vi "Miscellaneous_Initialization.vi"   [LabVIEW 2018]
uses:
  <vilib>/Rock Robotics/WPI/Joystick/WPI_JoystickDeviceEnum.ctl
  Subsytems/Drive/Drive_Notifier.ctl
  Subsytems/Drive/Drive_Control_Type.ctl
  Subsytems/Elevator/Elevator_Notifier.ctl
  Subsytems/Elevator/Elevator_Control_Type.ctl
  Subsytems/Elevator/Elevator_Enum_States.ctl
  Subsytems/Intake_Joint/Intake_Joint_Notifier.ctl
  Subsytems/Intake_Joint/Intake_Joint_Control_Type.ctl
  Subsytems/Intake_Joint/Intake_Joint_Enum_States.ctl
  Subsytems/Intake_Ball/Intake_Ball_Notifier.ctl
  Subsytems/Intake_Ball/Intake_Ball_Control_Type.ctl
  Subsytems/Intake_Disc/Intake_Disc_Notifier.ctl
  Subsytems/Intake_Disc/Intake_Disc_Control_Type.ctl
  <vilib>/Rock Robotics/WPI/Solenoid/WPI_SolenoidValue.ctl
  Subsytems/Climb/Climb_Notifier.ctl
  Subsytems/Climb/Climb_Control_Type.ctl
  <vilib>/Rock Robotics/SystemInterfaces/DIO/FPGA_DIOPWMChannel.ctl
  Global_Variables/Drive_Globals.vi
  Global_Variables/Refnum_Names.vi
  Global_Variables/Elevator_Globals.vi
  Global_Variables/Intake_Joint_Globals.vi
  Global_Variables/Intake_Ball_Globals.vi
  Global_Variables/Intake_Disc_Globals.vi
  Global_Variables/Climb_Globals.vi
  Global_Variables/LED_Globals.vi
types:
  T1 = typedef "FPGA_DIOPWMChannel.ctl" = enum8{"PWM 0", "PWM 1", "PWM 2", "PWM 3", "PWM 4", "PWM 5", "PWM 6", "PWM 7", "PWM 8", "PWM 9", "PWM MXP 0", "PWM MXP 1", "PWM MXP 2", "PWM MXP 3", "PWM MXP 4", "PWM MXP 5", "PWM MXP 6", "PWM MXP 7", "PWM MXP 8", "PWM MXP 9", "Invalid"}
  T2 = typedef "Climb_Notifier.ctl" = cluster{"Climb_Control_Type":T3, "Brake":bool, "Manual_Climb_Up":bool, "Manual_Drive_Forward":bool, "Manual_Drive_Backward":bool, "Manual_Climb_Down":bool, "Climb_Advance":bool, "Climb_Reverse":bool, "Parameter_One":dbl, "Parameter_Two":dbl, "Parameter_Three":dbl, "Step":i32, "Climb_Notifier":refnum<notifier>, "Climb_Distance":dbl, "Level_Two":bool, "Brake_State":bool, "Toggle_Servo":bool, "Drop_Back":bool}
  T3 = typedef "Climb_Control_Type.ctl" = enum16{"No_Op", "Brake", "Manual_Climb_Up", "Manual_Climb_Down", "Manual_Drive_Forward", "Manual_Drive_Backward", "Back_Wheels_Forward", "Lift_Retract", "Lift_Extend", "Extend_to_Second_Level", "Drop_Down", "Spin"}
  T4 = typedef "Intake_Disc_Notifier.ctl" = cluster{"Intake_Disc_Control_Type":T5, "Manual_Disc_Toggle":bool, "Disc_Toggle":bool, "Disc_Toggle_State":bool, "Manual_Press_Toggle":bool, "Disc_Press_State":bool, "Press_Toggle":bool, "Press_Pnuematic":T6, "Disc_Pnuematic":T6, "Disc_Notifier":refnum<notifier>, "Step":i32}
  T5 = typedef "Intake_Disc_Control_Type.ctl" = enum16{"No_Op", "Manual_Disc_Toggle", "Disc_Toggle", "Manual_Press_Toggle", "Press_Toggle", "Acquire_Hatch", "Retract"}
  T6 = typedef "WPI_SolenoidValue.ctl" = enum16{"Off", "On", "Forward", "Reverse"}
  T7 = typedef "Intake_Ball_Notifier.ctl" = cluster{"Intake_Ball_Control_Type":T8, "Manual_In":bool, "Manual_Out":bool, "Ball_In":bool, "Ball_Out":bool, "Parameter_One":dbl, "Parameter_Two":dbl, "Parameter_Three":dbl, "Step":i32, "Ball_Notifier":refnum<notifier>}
  T8 = typedef "Intake_Ball_Control_Type.ctl" = enum16{"No_Op", "Manual_In", "Manual_Out", "In_Sensor_Stop", "Out_Teleop", "Out", "Stall"}
  T9 = typedef "Intake_Joint_Notifier.ctl" = cluster{"Intake_Joint_Control_Type":T10, "Manual_Joint_Up":bool, "Manual_Joint_Down":bool, "Low_Rocket":bool, "Mid_Rocket":bool, "High_Rocket":bool, "Cargo_Ship":bool, "Hatch_Floor":bool, "Cargo_Floor":bool, "HP_Hatch":bool, "HP_Cargo":bool, "Depot_Cargo":bool, "Stow":bool, "Intake_Mode":bool, "Set Position":T11, "Parameter_One":dbl, "Parameter_Two":dbl, "Parameter_Three":dbl, "Step":i32, "Joint_Notifier":refnum<notifier>}
  T10 = typedef "Intake_Joint_Control_Type.ctl" = enum16{"No_Op", "Manual_Joint_Up", "Manual_Joint_Down", "Manual_Position_Control", "Position_Control", "Position"}
  T11 = typedef "Intake_Joint_Enum_States.ctl" = enum16{"Current_Position", "High_Rocket_Hatch_Panel_Floor", "High_Rocket_Hatch_Panel", "Mid_Rocket_Hatch_Panel_Floor", "Mid_Rocket_Hatch_Panel", "Low_Rocket_Hatch_Panel", "Cargo_Ship_Hatch_Panel", "Loading_Station_Hatch_Panel", "Ground_Pickup_Hatch_Panel", "High_Rocket_Cargo", "Mid_Rocket_Cargo", "Low_Rocket_Cargo", "Cargo_Ship_Cargo", "Loading_Station_Cargo", "Ground_Pickup_Cargo", "Depot_Pickup_Cargo", "Stow_Cargo", "Get_Hatch"}
  T12 = typedef "Elevator_Notifier.ctl" = cluster{"Elevator_Control_Type":T13, "Shift":bool, "Brake":bool, "Manual_Lift_Up":bool, "Manual_Lift_Down":bool, "Climb_Advance":bool, "Climb_Reverse":bool, "Low_Rocket":bool, "Mid_Rocket":bool, "High_Rocket":bool, "Cargo_Ship":bool, "Hatch_Floor":bool, "Cargo_Floor":bool, "HP_Hatch":bool, "HP_Cargo":bool, "Depot_Cargo":bool, "Stow":bool, "Set_Position":T14, "Intake_Mode":bool, "Climb_Distance":dbl, "Level_Two":bool, "Parameter_One":dbl, "Parameter_Two":dbl, "Parameter_Three":dbl, "Step":i32, "Elevator_Notifier":refnum<notifier>, "Brake_State":bool, "Shift_State":bool}
  T13 = typedef "Elevator_Control_Type.ctl" = enum16{"No_Op", "Shift", "Brake", "Manual_Elevator_Up", "Manual_Elevator_Down", "Manual_Climb_Up", "Manual_Climb_Down", "Manual_Position_Control", "Elevator_Retract", "Elevator_Extend", "Brake_In_Climb", "Position_Control", "Position", "Shift_Climb"}
  T14 = typedef "Elevator_Enum_States.ctl" = enum16{"Current_Position", "High_Rocket_Hatch_Panel_Floor", "High_Rocket_Hatch_Panel", "Mid_Rocket_Hatch_Panel_Floor", "Mid_Rocket_Hatch_Panel", "Low_Rocket_Hatch_Panel", "Cargo_Ship_Hatch_Panel", "Loading_Station_Hatch_Panel", "Ground_Pickup_Hatch_Panel", "High_Rocket_Cargo", "Mid_Rocket_Cargo", "Low_Rocket_Cargo", "Cargo_Ship_Cargo", "Loading_Station_Cargo", "Ground_Pickup_Cargo", "Depot_Pickup_Cargo", "Descend_Off_Platform", "Stow_Cargo"}
  T15 = typedef "Drive_Notifier.ctl" = cluster{"Drive Control List":T16, "Front/Back":dbl, "Left/Right":dbl, "Turn":dbl, "Test_Joy_Y":dbl, "Test_Joy_X":dbl, "Set Wheel Encoder Positions":bool, "Robotcentric":bool, "Reset Gyro":bool, "Rotate Front Right":bool, "Rotate Front Left":bool, "Rotate Back Right":bool, "Rotate Back Left":bool, "Write_Encoder_Positions":bool, "Climb_Advance":bool, "Parameter_One":dbl, "Parameter_Two":dbl, "Parameter_Three":dbl, "Parameter_Four":dbl, "Drive_Notifier":refnum<notifier>, "Step":i32, "Climb_Reverse":bool, "Auto_Target":bool}
  T16 = typedef "Drive_Control_Type.ctl" = enum16{"No_Op", "Write_FL_Position", "Write_FR_Position", "Write_BL_Position", "Write_BR_Position", "Set_Encoder_Positions", "Fieldcentric_PercentVBus", "Fieldcentric", "Robotcentric", "Reset_Gyro", "FR_Wheel", "FL_Wheel", "BR_Wheel", "BL_Wheel", "Drive_Onto_Platform", "Manual_Wheel_Control", "Distance", "Turn_To_Heading", "Turn_To_Target", "Drive_To_Target", "Zero", "Auto_Target", "Drive_Over_Platform", "Heading_Lock", "Time"}
  T17 = typedef "WPI_JoystickDeviceEnum.ctl" = enum16{"USB 0", "USB 1", "USB 2", "USB 3", "USB 4", "USB 5"}
  T18 = typedef "WPI_JoystickDevRef.ctl" = cluster{"Device":T17}
  T19 = typedef "CTRE_CANifier_DeviceRef.ctl" = cluster{"DeviceStatus":errorcluster, "Device Number":u8, "Handle":u64, "UsageFrame":u32, "Library Path":path}
  T20 = typedef "WPI_ServoDeviceRef.ctl" = cluster{"DeviceStatus":errorcluster, "PWM Channel":T1, "DeadBand":T21}
  T21 = typedef "WPI_PWMDeadband.ctl" = cluster{"Name":string, "maxPositivePwm":i32, "minPositivePwm":i32, "centerPwm":i32, "maxNegativePwm":i32, "minNegativePwm":i32, "angularRange":u16}
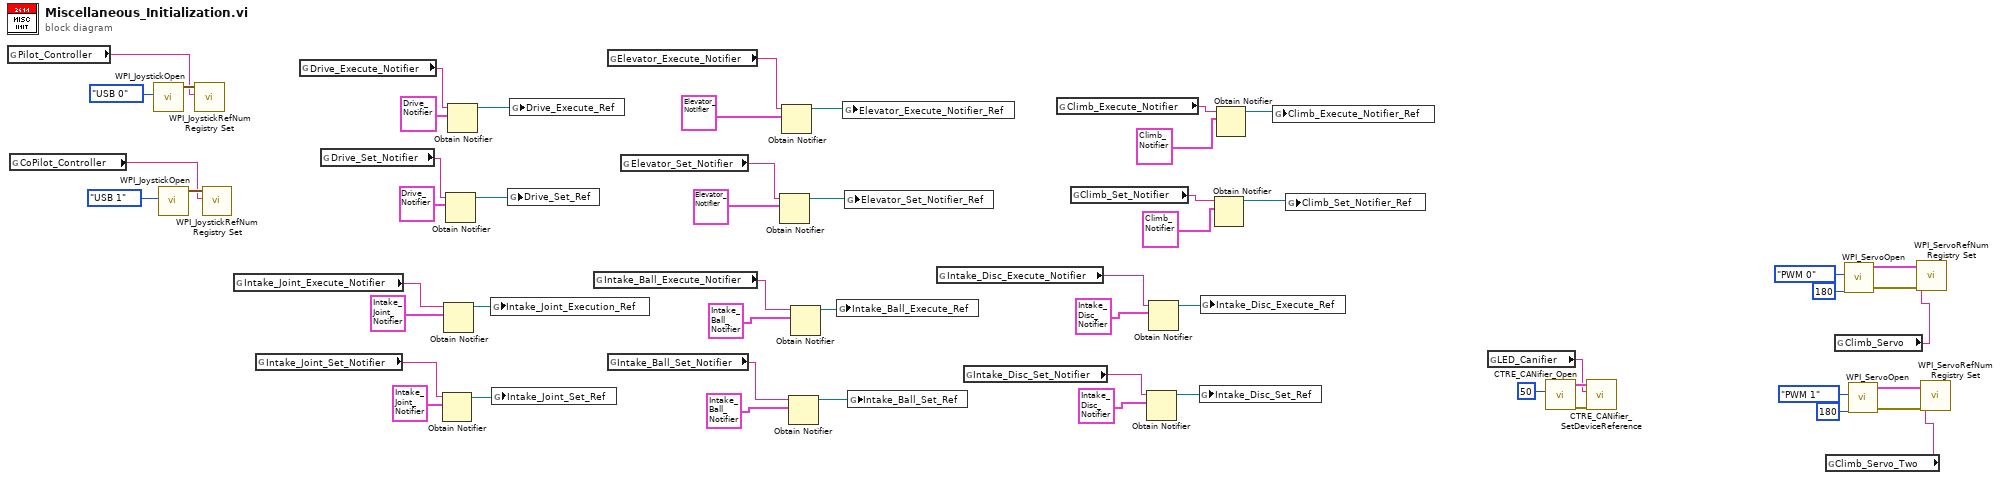
[diagram p0: block diagram]
diagram:
  n1 = global read "Refnum_Names.vi" "Pilot_Controller"() -> (w46:string)
  n2 = global read "Refnum_Names.vi" "CoPilot_Controller"() -> (w45:string)
  n3 = call <vilib>:"WPI_JoystickOpen.vi"("JoystickDevice"=WPI_JoystickDeviceEnum."USB 0") -> ("JoystickDevRef"=w56:T18)  [unwired: 10 in]
  n4 = call <vilib>:"WPI_JoystickOpen.vi"("JoystickDevice"=WPI_JoystickDeviceEnum."USB 1") -> ("JoystickDevRef"=w53:T18)  [unwired: 10 in]
  n5 = call <vilib>:"WPI_JoystickRefNum Registry Set.vi"("refnum name"=w46, "JoystickDevRef"=w56) -> ()  [unwired: 8 in, 2 out]
  n6 = call <vilib>:"WPI_JoystickRefNum Registry Set.vi"("refnum name"=w45, "JoystickDevRef"=w53) -> ()  [unwired: 8 in, 2 out]
  n7 = global read "Intake_Joint_Globals.vi" "Intake_Joint_Execute_Notifier"() -> (w36:string)
  n8 = global read "Intake_Joint_Globals.vi" "Intake_Joint_Set_Notifier"() -> (w35:string)
  n9 = global read "Drive_Globals.vi" "Drive_Execute_Notifier"() -> (w50:string)
  n10 = global read "Drive_Globals.vi" "Drive_Set_Notifier"() -> (w51:string)
  n11 = Obtain Notifier(name (unnamed)=w35, notification data type=T9 {"Intake_Joint_Control_Type"=enum."No_Op", "Manual_Joint_Up"=FALSE, "Manual_Joint_Down"=FALSE, "Low_Rocket"=FALSE, "Mid_Rocket"=FALSE, "High_Rocket"=FALSE, "Cargo_Ship"=FALSE, "Hatch_Floor"=FALSE, "Cargo_Floor"=FALSE, "HP_Hatch"=FALSE, "HP_Cargo"=FALSE, "Depot_Cargo"=FALSE, "Stow"=FALSE, "Intake_Mode"=FALSE, "Set Position"=enum."High_Rocket_Hatch_Panel", "Parameter_One"=0.0, "Parameter_Two"=0.0, "Parameter_Three"=0.0, "Step"=0, "Joint_Notifier"=refnum} ("Intake_Joint_Notifier")) -> (notifier out=w33:refnum<notifier>)  [unwired: 2 in, 2 out]
  n12 = Obtain Notifier(name (unnamed)=w36, notification data type=T9 {"Intake_Joint_Control_Type"=enum."No_Op", "Manual_Joint_Up"=FALSE, "Manual_Joint_Down"=FALSE, "Low_Rocket"=FALSE, "Mid_Rocket"=FALSE, "High_Rocket"=FALSE, "Cargo_Ship"=FALSE, "Hatch_Floor"=FALSE, "Cargo_Floor"=FALSE, "HP_Hatch"=FALSE, "HP_Cargo"=FALSE, "Depot_Cargo"=FALSE, "Stow"=FALSE, "Intake_Mode"=FALSE, "Set Position"=enum."High_Rocket_Hatch_Panel", "Parameter_One"=0.0, "Parameter_Two"=0.0, "Parameter_Three"=0.0, "Step"=0, "Joint_Notifier"=refnum} ("Intake_Joint_Notifier")) -> (notifier out=w34:refnum<notifier>)  [unwired: 2 in, 2 out]
  n13 = Obtain Notifier(name (unnamed)=w51, notification data type=T15 {"Drive Control List"=enum."No_Op", "Front/Back"=0.0, "Left/Right"=0.0, "Turn"=0.0, "Test_Joy_Y"=0.0, "Test_Joy_X"=0.0, "Set Wheel Encoder Positions"=FALSE, "Robotcentric"=FALSE, "Reset Gyro"=FALSE, "Rotate Front Right"=FALSE, "Rotate Front Left"=FALSE, "Rotate Back Right"=FALSE, "Rotate Back Left"=FALSE, "Write_Encoder_Positions"=FALSE, "Climb_Advance"=FALSE, "Parameter_One"=0.0, "Parameter_Two"=0.0, "Parameter_Three"=0.0, "Parameter_Four"=0.0, "Drive_Notifier"=refnum, "Step"=0, "Climb_Reverse"=FALSE, "Auto_Target"=FALSE} ("Drive Notifier")) -> (notifier out=w49:refnum<notifier>)  [unwired: 2 in, 2 out]
  n14 = Obtain Notifier(name (unnamed)=w50, notification data type=T15 {"Drive Control List"=enum."No_Op", "Front/Back"=0.0, "Left/Right"=0.0, "Turn"=0.0, "Test_Joy_Y"=0.0, "Test_Joy_X"=0.0, "Set Wheel Encoder Positions"=FALSE, "Robotcentric"=FALSE, "Reset Gyro"=FALSE, "Rotate Front Right"=FALSE, "Rotate Front Left"=FALSE, "Rotate Back Right"=FALSE, "Rotate Back Left"=FALSE, "Write_Encoder_Positions"=FALSE, "Climb_Advance"=FALSE, "Parameter_One"=0.0, "Parameter_Two"=0.0, "Parameter_Three"=0.0, "Parameter_Four"=0.0, "Drive_Notifier"=refnum, "Step"=0, "Climb_Reverse"=FALSE, "Auto_Target"=FALSE} ("Drive Notifier")) -> (notifier out=w52:refnum<notifier>)  [unwired: 2 in, 2 out]
  n15 = global write "Intake_Joint_Globals.vi" "Intake_Joint_Execution_Ref"(w34) -> ()
  n16 = global write "Intake_Joint_Globals.vi" "Intake_Joint_Set_Ref"(w33) -> ()
  n17 = global write "Drive_Globals.vi" "Drive_Set_Ref"(w49) -> ()
  n18 = global write "Drive_Globals.vi" "Drive_Execute_Ref"(w52) -> ()
  n19 = global read "Intake_Ball_Globals.vi" "Intake_Ball_Execute_Notifier"() -> (w32:string)
  n20 = global read "Elevator_Globals.vi" "Elevator_Execute_Notifier"() -> (w44:string)
  n21 = global read "Intake_Ball_Globals.vi" "Intake_Ball_Set_Notifier"() -> (w31:string)
  n22 = global read "Elevator_Globals.vi" "Elevator_Set_Notifier"() -> (w43:string)
  n23 = Obtain Notifier(name (unnamed)=w43, notification data type=T12 {"Elevator_Control_Type"=enum."No_Op", "Shift"=FALSE, "Brake"=FALSE, "Manual_Lift_Up"=FALSE, "Manual_Lift_Down"=FALSE, "Climb_Advance"=FALSE, "Climb_Reverse"=FALSE, "Low_Rocket"=FALSE, "Mid_Rocket"=FALSE, "High_Rocket"=FALSE, "Cargo_Ship"=FALSE, "Hatch_Floor"=FALSE, "Cargo_Floor"=FALSE, "HP_Hatch"=FALSE, "HP_Cargo"=FALSE, "Depot_Cargo"=FALSE, "Stow"=FALSE, "Set_Position"=enum."High_Rocket_Hatch_Panel", "Intake_Mode"=FALSE, "Climb_Distance"=0.0, "Level_Two"=FALSE, "Parameter_One"=0.0, "Parameter_Two"=0.0, "Parameter_Three"=0.0, "Step"=0, "Elevator_Notifier"=refnum, "Brake_State"=FALSE, "Shift_State"=FALSE} ("Elevator_Notifier")) -> (notifier out=w39:refnum<notifier>)  [unwired: 2 in, 2 out]
  n24 = Obtain Notifier(name (unnamed)=w44, notification data type=T12 {"Elevator_Control_Type"=enum."No_Op", "Shift"=FALSE, "Brake"=FALSE, "Manual_Lift_Up"=FALSE, "Manual_Lift_Down"=FALSE, "Climb_Advance"=FALSE, "Climb_Reverse"=FALSE, "Low_Rocket"=FALSE, "Mid_Rocket"=FALSE, "High_Rocket"=FALSE, "Cargo_Ship"=FALSE, "Hatch_Floor"=FALSE, "Cargo_Floor"=FALSE, "HP_Hatch"=FALSE, "HP_Cargo"=FALSE, "Depot_Cargo"=FALSE, "Stow"=FALSE, "Set_Position"=enum."High_Rocket_Hatch_Panel", "Intake_Mode"=FALSE, "Climb_Distance"=0.0, "Level_Two"=FALSE, "Parameter_One"=0.0, "Parameter_Two"=0.0, "Parameter_Three"=0.0, "Step"=0, "Elevator_Notifier"=refnum, "Brake_State"=FALSE, "Shift_State"=FALSE} ("Elevator_Notifier")) -> (notifier out=w40:refnum<notifier>)  [unwired: 2 in, 2 out]
  n25 = Obtain Notifier(name (unnamed)=w31, notification data type=T7 {"Intake_Ball_Control_Type"=enum."No_Op", "Manual_In"=FALSE, "Manual_Out"=FALSE, "Ball_In"=FALSE, "Ball_Out"=FALSE, "Parameter_One"=0.0, "Parameter_Two"=0.0, "Parameter_Three"=0.0, "Step"=0, "Ball_Notifier"=refnum} ("Intake_Ball_Notifier")) -> (notifier out=w27:refnum<notifier>)  [unwired: 2 in, 2 out]
  n26 = Obtain Notifier(name (unnamed)=w32, notification data type=T7 {"Intake_Ball_Control_Type"=enum."No_Op", "Manual_In"=FALSE, "Manual_Out"=FALSE, "Ball_In"=FALSE, "Ball_Out"=FALSE, "Parameter_One"=0.0, "Parameter_Two"=0.0, "Parameter_Three"=0.0, "Step"=0, "Ball_Notifier"=refnum} ("Intake_Ball_Notifier")) -> (notifier out=w28:refnum<notifier>)  [unwired: 2 in, 2 out]
  n27 = global write "Intake_Ball_Globals.vi" "Intake_Ball_Execute_Ref"(w28) -> ()
  n28 = global write "Elevator_Globals.vi" "Elevator_Execute_Notifier_Ref"(w40) -> ()
  n29 = global write "Elevator_Globals.vi" "Elevator_Set_Notifier_Ref"(w39) -> ()
  n30 = global write "Intake_Ball_Globals.vi" "Intake_Ball_Set_Ref"(w27) -> ()
  n31 = global read "Intake_Disc_Globals.vi" "Intake_Disc_Execute_Notifier"() -> (w24:string)
  n32 = global read "Intake_Disc_Globals.vi" "Intake_Disc_Set_Notifier"() -> (w23:string)
  n33 = global read "Climb_Globals.vi" "Climb_Execute_Notifier"() -> (w19:string)
  n34 = global read "Climb_Globals.vi" "Climb_Set_Notifier"() -> (w20:string)
  n35 = Obtain Notifier(name (unnamed)=w23, notification data type=T4 {"Intake_Disc_Control_Type"=enum."No_Op", "Manual_Disc_Toggle"=FALSE, "Disc_Toggle"=FALSE, "Disc_Toggle_State"=FALSE, "Manual_Press_Toggle"=FALSE, "Disc_Press_State"=FALSE, "Press_Toggle"=FALSE, "Press_Pnuematic"=enum."Forward", "Disc_Pnuematic"=enum."Forward", "Disc_Notifier"=refnum, "Step"=0} ("Intake_Disc_Notifier")) -> (notifier out=w21:refnum<notifier>)  [unwired: 2 in, 2 out]
  n36 = Obtain Notifier(name (unnamed)=w24, notification data type=T4 {"Intake_Disc_Control_Type"=enum."No_Op", "Manual_Disc_Toggle"=FALSE, "Disc_Toggle"=FALSE, "Disc_Toggle_State"=FALSE, "Manual_Press_Toggle"=FALSE, "Disc_Press_State"=FALSE, "Press_Toggle"=FALSE, "Press_Pnuematic"=enum."Forward", "Disc_Pnuematic"=enum."Forward", "Disc_Notifier"=refnum, "Step"=0} ("Intake_Disc_Notifier")) -> (notifier out=w22:refnum<notifier>)  [unwired: 2 in, 2 out]
  n37 = global write "Intake_Disc_Globals.vi" "Intake_Disc_Set_Ref"(w21) -> ()
  n38 = global write "Intake_Disc_Globals.vi" "Intake_Disc_Execute_Ref"(w22) -> ()
  n39 = Obtain Notifier(name (unnamed)=w20, notification data type=T2 {"Climb_Control_Type"=enum."No_Op", "Brake"=FALSE, "Manual_Climb_Up"=FALSE, "Manual_Drive_Forward"=FALSE, "Manual_Drive_Backward"=FALSE, "Manual_Climb_Down"=FALSE, "Climb_Advance"=FALSE, "Climb_Reverse"=FALSE, "Parameter_One"=0.0, "Parameter_Two"=0.0, "Parameter_Three"=0.0, "Step"=0, "Climb_Notifier"=refnum, "Climb_Distance"=0.0, "Level_Two"=FALSE, "Brake_State"=FALSE, "Toggle_Servo"=FALSE, "Drop_Back"=FALSE} ("Climb_Notifier")) -> (notifier out=w17:refnum<notifier>)  [unwired: 2 in, 2 out]
  n40 = Obtain Notifier(name (unnamed)=w19, notification data type=T2 {"Climb_Control_Type"=enum."No_Op", "Brake"=FALSE, "Manual_Climb_Up"=FALSE, "Manual_Drive_Forward"=FALSE, "Manual_Drive_Backward"=FALSE, "Manual_Climb_Down"=FALSE, "Climb_Advance"=FALSE, "Climb_Reverse"=FALSE, "Parameter_One"=0.0, "Parameter_Two"=0.0, "Parameter_Three"=0.0, "Step"=0, "Climb_Notifier"=refnum, "Climb_Distance"=0.0, "Level_Two"=FALSE, "Brake_State"=FALSE, "Toggle_Servo"=FALSE, "Drop_Back"=FALSE} ("Climb_Notifier")) -> (notifier out=w18:refnum<notifier>)  [unwired: 2 in, 2 out]
  n41 = global write "Climb_Globals.vi" "Climb_Execute_Notifier_Ref"(w18) -> ()
  n42 = global write "Climb_Globals.vi" "Climb_Set_Notifier_Ref"(w17) -> ()
  n43 = global read "LED_Globals.vi" "LED_Canifier"() -> (w11:string)
  n44 = call <vilib>:"CTRE_CANifier_Open.vi"("Device Number"=u8 50) -> ("error out"=w13:errorcluster, "CANifierDevRef"=w12:T19)  [unwired: 9 in]
  n45 = call <vilib>:"CTRE_CANifier_SetDeviceReference.vi"("error in (no error)"=w13, "refnum name"=w11, "CANifierDevRef"=w12) -> ()  [unwired: 7 in, 2 out]
  n46 = global read "Climb_Globals.vi" "Climb_Servo_Two"() -> (w5:string)
  n47 = global read "Climb_Globals.vi" "Climb_Servo"() -> (w6:string)
  n48 = call <vilib>:"WPI_ServoOpen.vi"("Angular Range"=u16 180, "PWM Channel"=FPGA_DIOPWMChannel."PWM 0") -> ("error out"=w9:errorcluster, "ServoDeviceRef"=w10:T20)  [unwired: 8 in]
  n49 = call <vilib>:"WPI_ServoOpen.vi"("Angular Range"=u16 180, "PWM Channel"=FPGA_DIOPWMChannel."PWM 1") -> ("error out"=w2:errorcluster, "ServoDeviceRef"=w1:T20)  [unwired: 8 in]
  n50 = call <vilib>:"WPI_ServoRefNum Registry Set.vi"("error in (no error)"=w9, "refnum name"=w6, "ServoDeviceRef"=w10) -> ()  [unwired: 7 in, 2 out]
  n51 = call <vilib>:"WPI_ServoRefNum Registry Set.vi"("error in (no error)"=w2, "refnum name"=w5, "ServoDeviceRef"=w1) -> ()  [unwired: 7 in, 2 out]
